vi "increment,decrementevent.vi"() -> ()   [LabVIEW 2018]
panel:
  in  "stop":bool
  out "x+1":dbl
  in  "Decrement":bool
  in  "Increment":bool
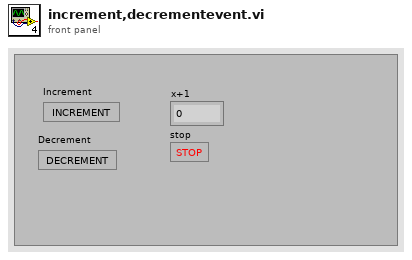
[diagram p1: front panel]
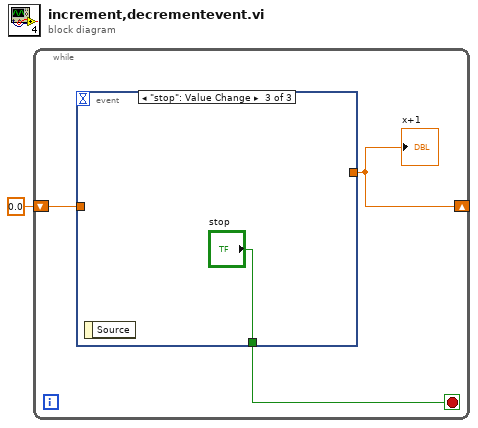
[diagram p0: block diagram]
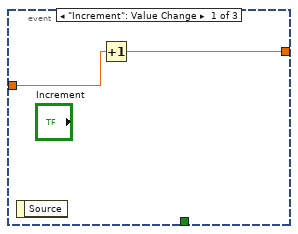
[diagram p2: hidden frame]
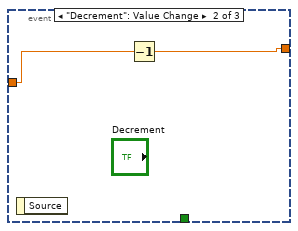
[diagram p3: hidden frame]
diagram:
  n1 = while {
    shift-right: [w3] -> _
    shift-left: 0.0 -> [w4]
    stop <- w2 stop-if-true
    n2 = event shown="[2] \"stop\": Value Change" {
      selector: _ -> [_ _ _]
      dyn-events: _ -> [_ _ _]
      timeout: _ -> [_ _ _]
      tunnel: [w6 w7 _] -> w3
      tunnel: w4 -> [w5 w8 _]
      tunnel: [_ _ "stop"] -> w2
      event "Increment": Value Change {
        n3 = event-data() -> ()  [unwired: 1 in, 1 out]
        n4 = Increment(x=w5) -> (x+1=w6:dbl)
      }
      event "Decrement": Value Change {
        n5 = event-data() -> ()  [unwired: 1 in, 1 out]
        n6 = Decrement(x=w8) -> (x-1=w7:dbl)
      }
      event "stop": Value Change {
        n7 = event-data() -> ()  [unwired: 1 in, 1 out]
      }
    }
    "x+1" <- w3
  }
